vi "Test Load ECM Profile.vi"() -> ()   [LabVIEW 2023]
uses:
  <vilib>/Python/Open Venv Python Session.vi
panel:
  out "XY Graph":cluster{"X":dbl, "Y":dbl}[](graph)
  out "value":dbl[][](array[numeric])
  out "ocv_soc_profile":string
  out "profile loaded":bool
  in  "module path":path=path "hps17k-pybamm-wrapper.py"
  out "error out":errorcluster
  in  "Env path":path
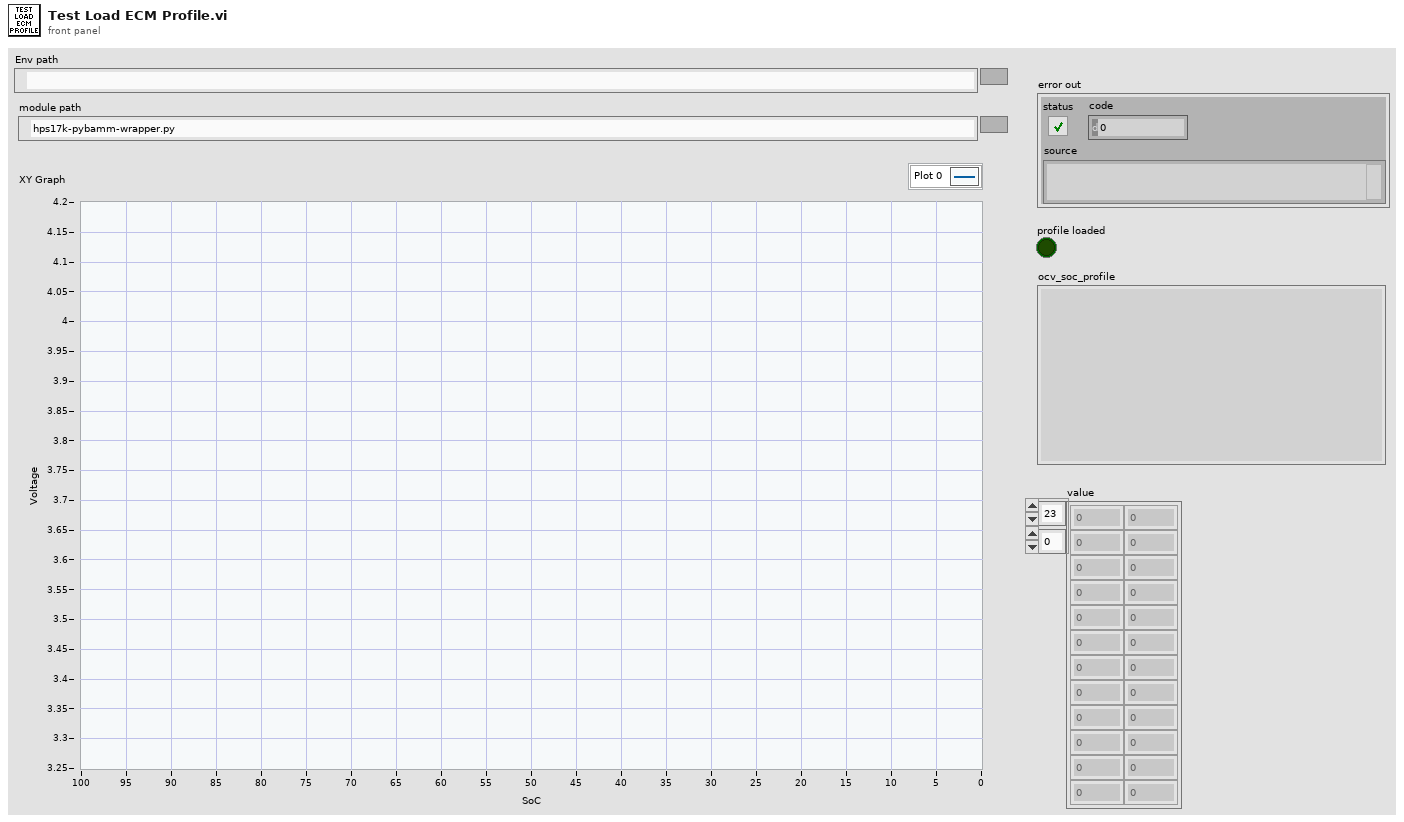
[diagram p1: front panel]
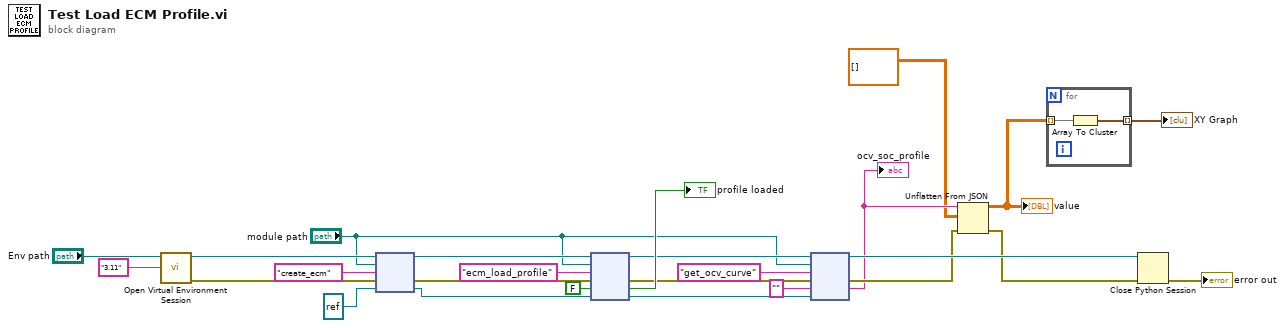
[diagram p0: block diagram]
diagram:
  n1 = call-poly <vilib>:"Open Virtual Environment Session.vi"("Python version"="3.11", "Env path"="Env path") -> ("error out"=w26:errorcluster, "session out"=w25:refnum<k35>)  [unwired: 8 in]
  n2 = node(w25, "module path", "create_ecm" ("function name"), w26, refnum<k38> refnum ("Python Object Refnum")) -> (w19:refnum<k35>, w18:errorcluster, w8:refnum<k38>)  [unwired: 2 out]
  n3 = node(w19, "module path", "ecm_load_profile" ("function name"), w18, FALSE, w8) -> (w14:refnum<k35>, w13:errorcluster, →"profile loaded":bool, w7:refnum<k38>)  [unwired: 2 out]
  n4 = node(w14, "module path", "get_ocv_curve" ("function name"), w13, "", w7) -> (w12:refnum<k35>, w6:errorcluster, w4:string)  [unwired: 1 in, 2 out]
  "ocv_soc_profile" <- w4
  n5 = Unflatten From JSON(JSON string=w4, type and defaults=dbl[][] [], error in (no error)=w6) -> (value=w2:dbl[][], error out=w5:errorcluster)  [unwired: 4 in]
  "value" <- w2
  n6 = for {
    tunnel: w2 -> [w28] mode=indexing
    tunnel: [w27] -> w1 mode=indexing
    n7 = Array To Cluster(array=w28) -> (cluster=w27:cluster{"[0]":dbl, "[1]":dbl})
  }
  "XY Graph" <- w1
  n8 = Close Python Session(session in=w12, error in=w5) -> (11:→"error out":errorcluster)
